vi "Convert Path.vi"(8 "error in (no error)":errorcluster, 10 "Target OS":enum16{"Pharlap", "VxWorks"}(ring), 11 "Path in":path) -> (0 "error out":errorcluster, 2 "Formatted Path":string, 3 "Path out":path)   [LabVIEW 2016, in "Scan Engine Custom Device.lvlib"]
uses:
  Scan Engine Custom Device.lvlib
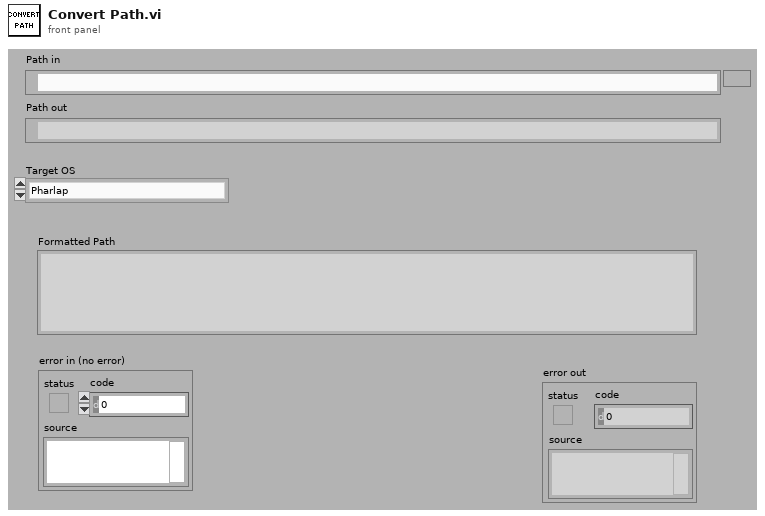
[diagram p1: front panel]
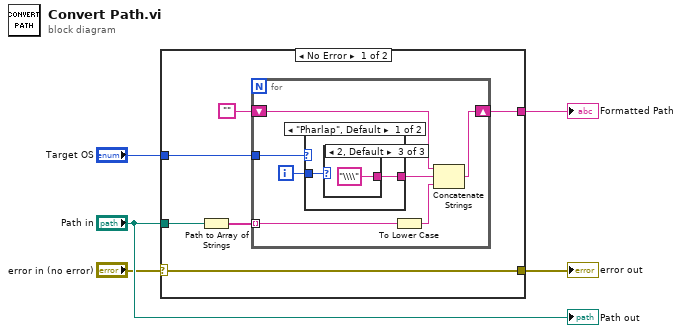
[diagram p0: block diagram]
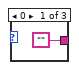
[diagram p2: hidden frame]
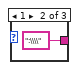
[diagram p3: hidden frame]
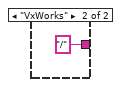
[diagram p4: hidden frame]
diagram:
  n1 = case shown="No Error" "error in (no error)" {
    selector: "error in (no error)" -> [w6 w25]
    tunnel: "Path in" -> [w11 _]
    tunnel: [w9 _] -> w4
    tunnel: "Target OS" -> [w7 _]
    tunnel: [w6 w25] -> w1
    frame No Error {
      n2 = Path to Array of Strings(0:w11) -> (2:w10:string[])  [unwired: 1 out]
      n3 = for {
        tunnel: w10 -> [w16] mode=indexing
        shift-right: [w17] -> w9
        shift-left: "" -> [w18]
        tunnel: w7 -> [w15]
        i -> [w14]
        n4 = case shown="\"Pharlap\", Default" w15 {
          tunnel: w14 -> [w20 _]
          tunnel: [w19 "/"] -> w12
          frame "Pharlap", Default {
            n5 = case shown="2, Default" w20 {
              tunnel: ["" ":\\\\" "\\\\"] -> w19
              frame 0 {
              }
              frame 1 {
              }
              frame 2, Default {
              }
            }
          }
          frame "VxWorks" {
          }
        }
        n6 = To Lower Case(string=w16) -> (all lower case string=w13:string)
        n7 = Concatenate Strings(w18, w12, w13) -> (w17:string)
      }
    }
    frame Error {
    }
  }
  "Formatted Path" <- w4
  "error out" <- w1
  "Path out" <- "Path in"
